vi "Add Block Diagram Content.vi"(8 "error in (no error)":errorcluster, 10 "ModuleLoop":T1, 11 "FPGA Addon Output in":refnum<class "FPGA Addon Output.lvclass">) -> (0 "error out":errorcluster, 2 "Term Refnum":refnum<vi>, 3 "FPGA Addon Output out":refnum<class "FPGA Addon Output.lvclass">)   [LabVIEW 2015, in "FPGA Addon Output.lvclass"]
uses:
  FPGA Addon Output.lvclass
  Loop/Block Diagram/Module.Refs.ctl
  <vilib>/Utility/miscctls.llb/LVPointTypeDef.ctl
  SubVIs/FPGAAddon.SpecialityOutputs.Generate.Parameters.ctl
  Loop/Structures/Structures.lvclass
  Loop/Block Diagram/Block Diagram.lvclass
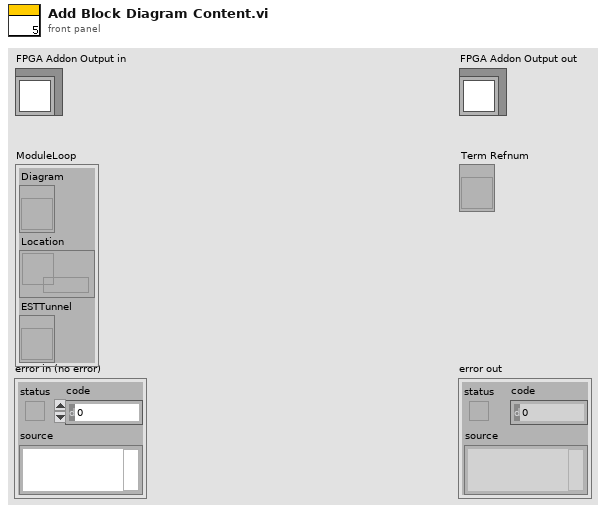
[diagram p1: front panel]
types:
  T1 = typedef "Block Diagram.lvclass/Module.Refs.ctl" = cluster{"Diagram":refnum<vi>, "Location":refnum<data-value>, "ESTTunnel":refnum<vi>}
  T2 = typedef "FPGAAddon.SpecialityOutputs.Generate.Parameters.ctl" = cluster{"Parent":refnum<vi>, "subVI path":path, "location":T3, "IO Name":string}
  T3 = typedef "LVPointTypeDef.ctl" = cluster{"Horizontal":i16, "Vertical":i16}
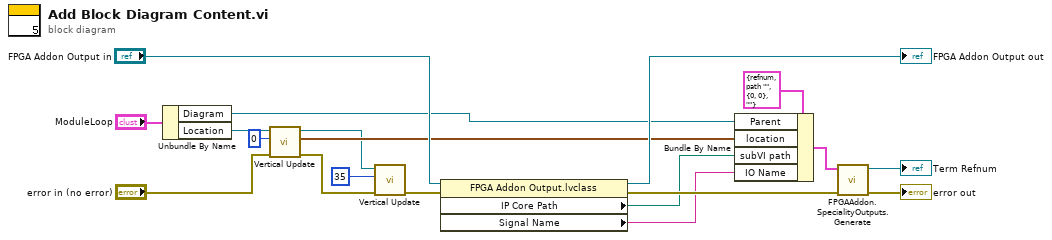
[diagram p0: block diagram]
diagram:
  n1 = Unbundle By Name("ModuleLoop") -> ("Diagram"=w1:refnum<vi>, "Location"=w7:refnum<data-value>)
  n2 = call "Vertical Update.vi"("error in (no error)"="error in (no error)", "Vertical Change"=i16 0, "Location"=w7) -> ("error out"=w3:errorcluster, "location out"=w9:T3, "Location"=w5:refnum<data-value>)  [unwired: 6 in]
  n3 = call "Vertical Update.vi"("error in (no error)"=w3, "Vertical Change"=i16 35, "Location"=w5) -> ("error out"=w2:errorcluster)  [unwired: 6 in, 2 out]
  n4 = property class="FPGA Addon Output.lvclass"(reference="FPGA Addon Output in", error in=w2) -> (reference out=→"FPGA Addon Output out":refnum<class "FPGA Addon Output.lvclass">, error out=w14:errorcluster, "IP Core Path"=w13:path, "Signal Name"=w12:string)
  n5 = Bundle By Name(cluster=T2 {"Parent"=refnum, "subVI path"=path "", "location"={"Horizontal"=0, "Vertical"=0}, "IO Name"=""} ("Parameters"), "Parent"=w1, "location"=w9, "subVI path"=w13, "IO Name"=w12) -> (w18:T2)
  n6 = call "FPGAAddon.SpecialityOutputs.Generate.vi"("error in (no error)"=w14, "Parameters"=w18) -> ("error out"=→"error out":errorcluster, "Output.Ref"=→"Term Refnum":refnum<vi>)  [unwired: 8 in]
